vi "Gaussians with offset model.vi"(3 "output control":T1, 4 "data":variant, 5 "X":dbl[](array[numeric]), 6 "a":dbl[](array[numeric])) -> (0 "error out":errorcluster, 1 "f'(X,a)":dbl[][](array[numeric]), 2 "f(X,a)":dbl[](array[numeric]))   [LabVIEW 2020]
doc: "Sum of three Gaussians, plus DC offset."
uses:
  <vilib>/gmath/NumericalOptimization/LM_output select.ctl
  <vilib>/gmath/NI_Gmath.lvlib
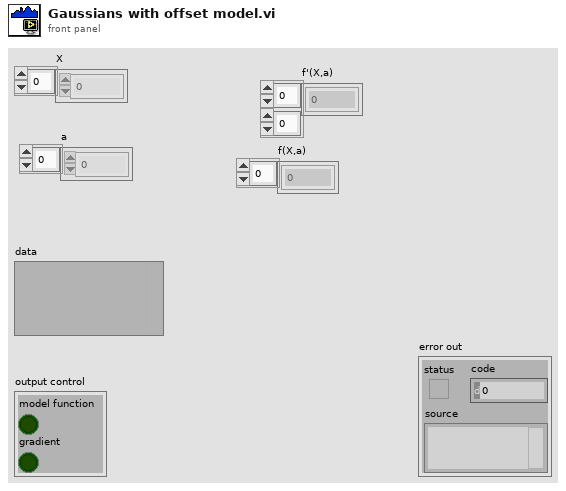
[diagram p1: front panel]
types:
  T1 = typedef "NI_Gmath.lvlib/LM_output select.ctl" = cluster{"model function":bool, "gradient":bool}
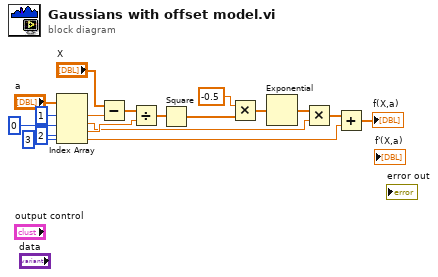
[diagram p0: block diagram]
diagram:
  n1 = Index Array(array="a", index #1=1 ("index"), index #2=0 ("index"), index #3=2 ("index"), index #4=3 ("index")) -> (element #1=w16:dbl, element #2=w8:dbl, element #3=w14:dbl, element #4=w6:dbl)
  n2 = Subtract(x="X", y=w16) -> (x-y=w15:dbl[])
  n3 = Divide(x=w15, y=w14) -> (x/y=w13:dbl[])
  n4 = Square(x=w13) -> (x^2=w12:dbl[])
  n5 = Multiply(x=-0.5, y=w12) -> (x*y=w10:dbl[])
  n6 = Exponential(1:w10) -> (0:w9:dbl[])
  n7 = Multiply(x=w9, y=w8) -> (x*y=w7:dbl[])
  n8 = Add(x=w7, y=w6) -> (x+y=→"f(X,a)":dbl[])
